vi "New.vi"(8 "error in (no error)":errorcluster, 11 "reference in":refnum<class "TestSuite_InterfaceDelegation.lvclass">) -> (0 "error out":errorcluster, 3 "reference out":refnum<class "TestSuite_InterfaceDelegation.lvclass">)   [LabVIEW 2009, in "TestSuite_InterfaceDelegation.lvclass"]
uses:
  TestSuite_InterfaceDelegation.lvclass
  Test Cases/List_Delegations/List_Delegations.lvclass
  Test Cases/StringList_Delegations/StringList_Delegations.lvclass
  <vilib>/addons/_JKI Toolkits/VI Tester/TestCase.llb/TestCase.lvclass
  TestSuite_InterfaceDelegation.lvclass/TestSuite_InterfaceDelegation.ctl
  <vilib>/addons/_JKI Toolkits/VI Tester/TestSuite.llb/TestSuite.lvclass
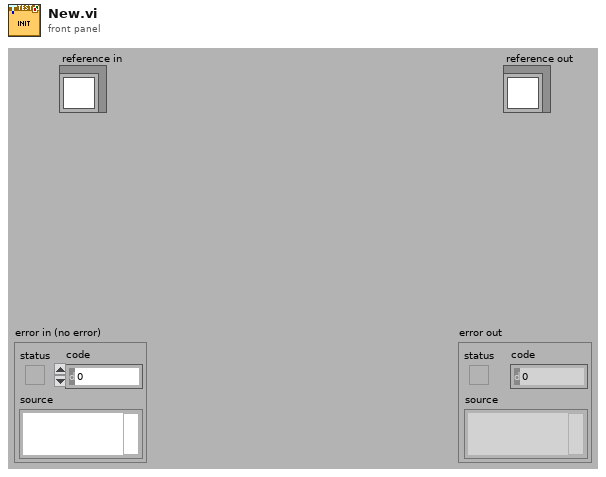
[diagram p1: front panel]
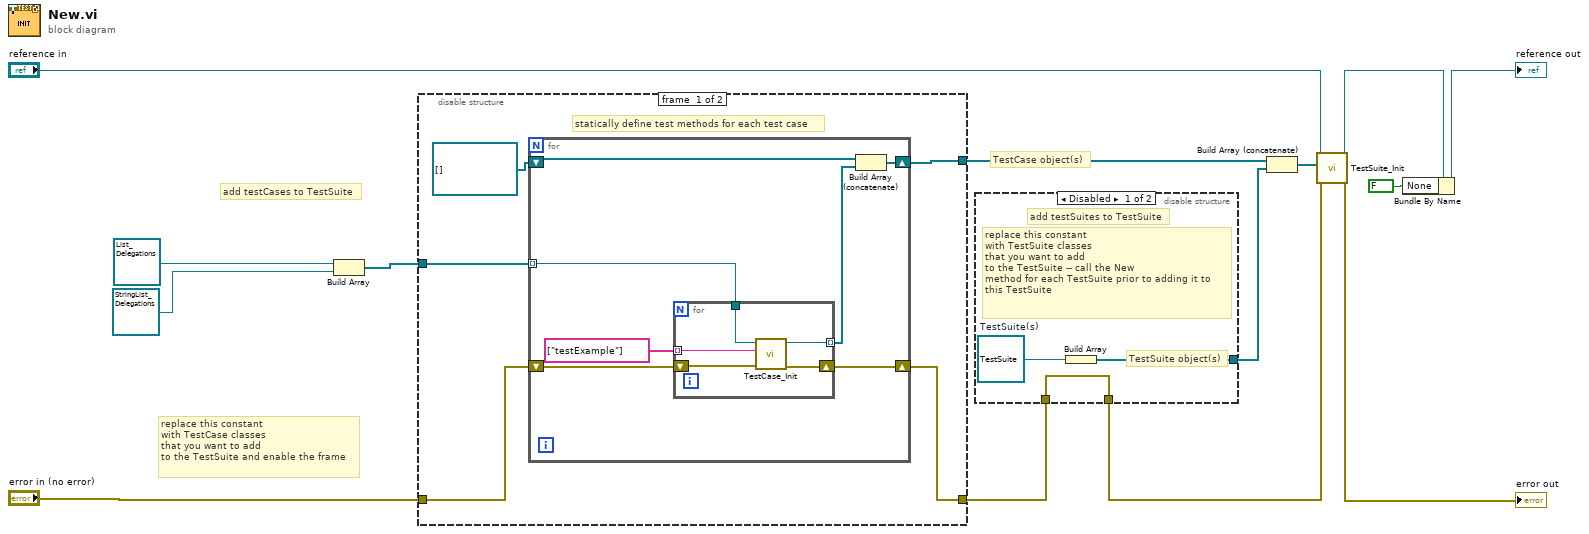
[diagram p0: block diagram]
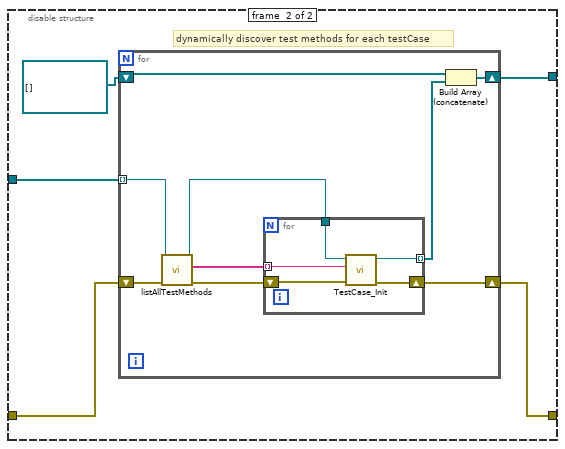
[diagram p3: hidden frame]
diagram:
  # "replace this constant\nwith TestCase classes\nthat you want to add\nto the TestSuite and enable the frame"
  # "TestCase object(s)"
  # "add testCases to TestSuite"
  n1 = Build Array(refnum<class "List_Delegations.lvclass"> refnum ("List_Delegations.lvclass"), refnum<class "StringList_Delegations.lvclass"> refnum ("StringList_Delegations.lvclass")) -> (w8:refnum<class "TestCase.lvclass">[])
  n2 = disable-structure shown="Enabled" {
    disable-tunnel: w8 -> [w19 w36]
    disable-tunnel: "error in (no error)" -> [w17 w34]
    disable-tunnel: [w16 w33] -> w7
    disable-tunnel: [w15 w32] -> w3
    frame #0 {
      # "statically define test methods for each test case"
      n3 = for {
        shift-right: [w24] -> w15
        shift-left: w17 -> [w25]
        tunnel: w19 -> [w23] mode=indexing
        shift-right: [w20] -> w16
        shift-left: refnum<class "TestCase.lvclass">[] [] -> [w21]
        n4 = for {
          tunnel: w23 -> [w27]
          tunnel: string[] ["testExample"] ("tests") -> [w31] mode=indexing
          shift-right: [w29] -> w24
          shift-left: w25 -> [w30]
          tunnel: [w28] -> w22 mode=indexing
          n5 = call <vilib>:"TestCase_Init.vi"("error in (no error)"=w30, "methodName (\"runTest\")"=w31, "TestCase in"=w27) -> ("error out"=w29:errorcluster, "TestCase out"=w28:refnum<class "TestCase.lvclass">)  [unwired: 7 in]
        }
        n6 = Build Array (concatenate)(w21, w22) -> (w20:refnum<class "TestCase.lvclass">[])
      }
    }
    frame #1 {
      # "dynamically discover test methods for each testCase"
      n7 = for {
        shift-right: [w45] -> w32
        shift-left: w34 -> [w41]
        tunnel: w36 -> [w38] mode=indexing
        shift-right: [w42] -> w33
        shift-left: refnum<class "TestCase.lvclass">[] [] -> [w43]
        n8 = call-dynamic "listAllTestMethods.vi"("error in (no error)"=w41, "TestCase in"=w38) -> ("error out"=w40:errorcluster, "test methods"=w39:string[], "TestCase out"=w37:refnum<class "TestCase.lvclass">)  [unwired: 7 in]
        n9 = for {
          tunnel: w37 -> [w46]
          tunnel: w39 -> [w50] mode=indexing
          shift-right: [w48] -> w45
          shift-left: w40 -> [w49]
          tunnel: [w47] -> w44 mode=indexing
          n10 = call <vilib>:"TestCase_Init.vi"("error in (no error)"=w49, "methodName (\"runTest\")"=w50, "TestCase in"=w46) -> ("error out"=w48:errorcluster, "TestCase out"=w47:refnum<class "TestCase.lvclass">)  [unwired: 7 in]
        }
        n11 = Build Array (concatenate)(w43, w44) -> (w42:refnum<class "TestCase.lvclass">[])
      }
    }
  }
  n12 = disable-structure shown="Disabled" {
    disable-tunnel: [w51 _] -> w5
    disable-tunnel: [w53 w54] -> w4
    disable-tunnel: w3 -> [w53 w54]
    frame #0 {
      w52 = refnum<class "TestSuite.lvclass"> refnum  # TestSuite(s)
      # "replace this constant\nwith TestSuite classes\nthat you want to add\nto the TestSuite -- call the New\nmethod for each TestSuite prior to adding it to\nthis TestSuite"
      # "add testSuites to TestSuite"
      # "TestSuite object(s)"
      n13 = Build Array(w52) -> (w51:refnum<class "TestSuite.lvclass">[])
    }
    frame #1 {
    }
  }
  n14 = Build Array (concatenate)(w7, w5) -> (w6:refnum<class>[])
  n15 = call <vilib>:"TestSuite_Init.vi"("error in (no error)"=w4, "tests (none)"=w6, "TestSuite in"="reference in") -> ("error out"=→"error out":errorcluster, "TestSuite out"=w9:refnum<class "TestSuite_InterfaceDelegation.lvclass">)  [unwired: 7 in]
  n16 = Bundle By Name(cluster=w9, "None"=FALSE) -> (→"reference out":refnum<class "TestSuite_InterfaceDelegation.lvclass">)
